vi "Filter.vi"(8 "error in (no error)":errorcluster, 10 "Test Suite":refnum<class "LUnit Test Suite.lvclass">, 11 "Inherited Tests Filter In":refnum<class "Inherited Tests Filter.lvclass">) -> (0 "error out":errorcluster, 2 "Filtered Test Suite":refnum<class "LUnit Test Suite.lvclass">)   [LabVIEW 2020, in "Inherited Tests Filter.lvclass"]
uses:
  Inherited Tests Filter.lvclass
  API/LUnit Test Suite/LUnit Test Suite.lvclass
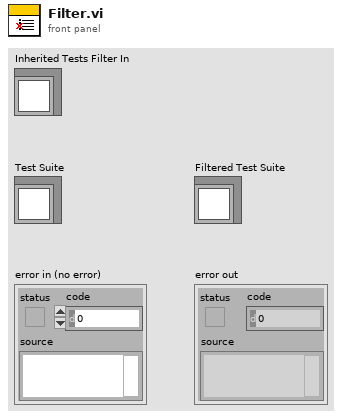
[diagram p1: front panel]
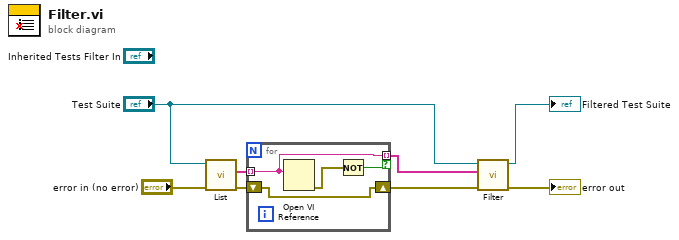
[diagram p0: block diagram]
diagram:
  n1 = call "List.vi"("error in (no error)"="error in (no error)", "LUnit Test Suite In"="Test Suite") -> ("error out"=w6:errorcluster, "List of Runnables"=w7:string[])  [unwired: 8 in]
  n2 = for {
    tunnel: w7 -> [w12] mode=indexing
    tunnel: [w12] -> w8 mode=indexing if=w10
    shift-right: [w9] -> w5
    shift-left: w6 -> [w9]
    n3 = Open VI Reference(vi path=w12) -> (error out=w11:errorcluster)  [unwired: 5 in, 1 out]
    n4 = Not(x=w11) -> (.not. x?=w10:bool)
  }
  n5 = call "Filter.vi"("error in (no error)"=w5, "Selected Runnables"=w8, "LUnit Test Suite In"="Test Suite") -> ("error out"=→"error out":errorcluster, "LUnit Test Suite Out"=→"Filtered Test Suite":refnum<class "LUnit Test Suite.lvclass">)  [unwired: 7 in]
